vi "Polynomial Roots (DBL).vi"(10 "option":u16(ring)=1 items=["General", "Simple Classification", "Refinement", "Advanced Refinement"], 11 "P(x)":dbl[](array[numeric])) -> (0 "error":i32, 3 "Roots":cdb[](array[numeric]))   [LabVIEW 2020, in "NI_AALPro.lvlib"]
doc: "Finds the roots of polynomial <B>P(x)</B>. This VI removes leading coefficients of the polynomial that are equal to zero. Wire data to the <B>P(x)</B> input to determine the polymorphic instance to use or manually select the instance."
uses:
  NI_AALPro.lvlib
  <resource>/lvanlys.dll
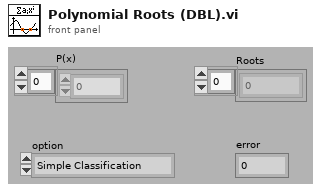
[diagram p1: front panel]
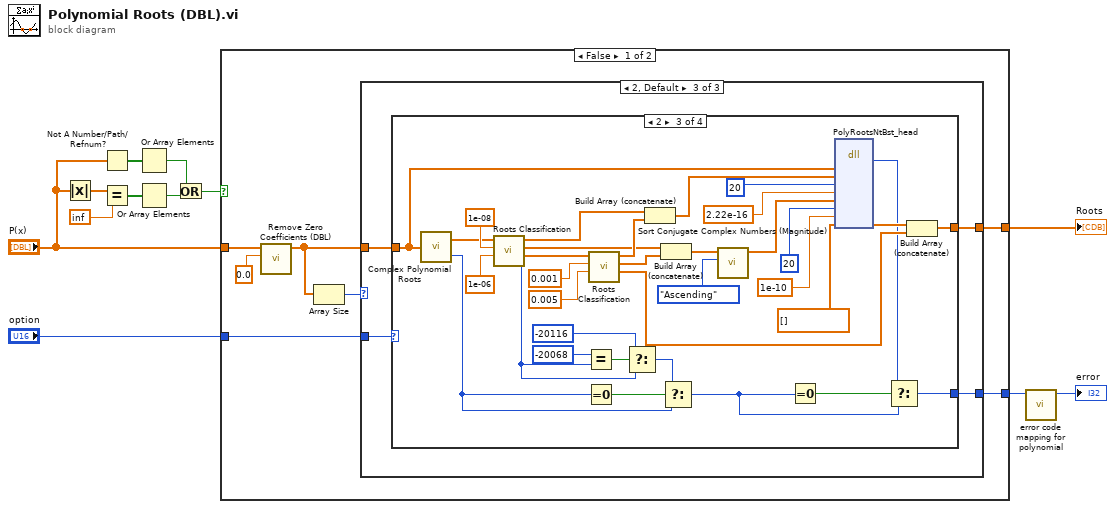
[diagram p0: block diagram]
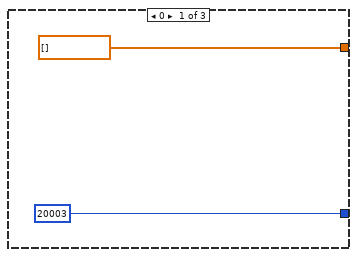
[diagram p2: hidden frame]
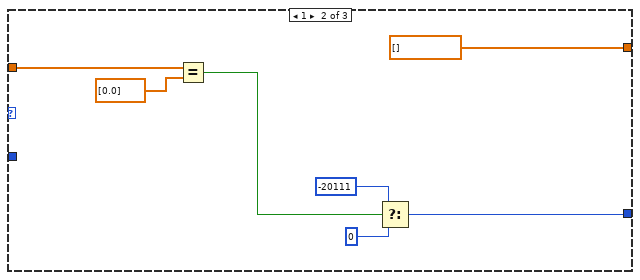
[diagram p3: hidden frame]
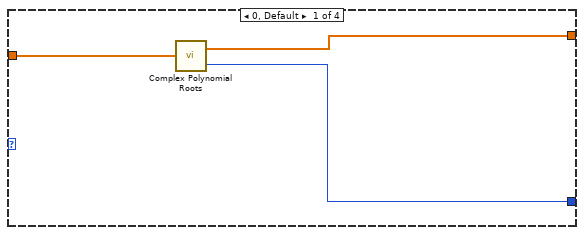
[diagram p4: hidden frame]
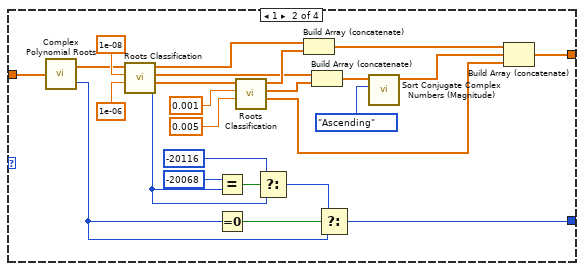
[diagram p5: hidden frame]
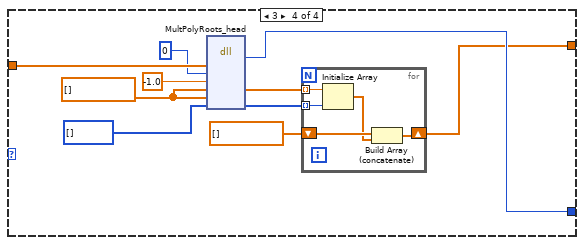
[diagram p6: hidden frame]
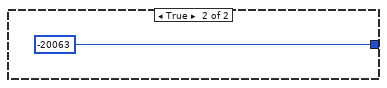
[diagram p7: hidden frame]
diagram:
  n1 = Absolute Value(x="P(x)") -> (abs(x)=w7:dbl[])
  n2 = Not A Number/Path/Refnum?(number/path/refnum="P(x)") -> (NaN/Path/Refnum?=w8:bool[])
  n3 = Equal?(x=w7, y=inf) -> (x = y?=w5:bool[])
  n4 = Or Array Elements(Boolean array=w8) -> (logical OR=w4:bool)
  n5 = Or Array Elements(Boolean array=w5) -> (logical OR=w3:bool)
  n6 = Or(x=w4, y=w3) -> (x .or. y?=w1:bool)
  n7 = case shown="False" w1 {
    tunnel: [w19 _] -> w12
    tunnel: "option" -> [w17 _]
    tunnel: [w16 -20063 ("error")] -> w10
    tunnel: "P(x)" -> [w14 _]
    frame False {
      n8 = call "Remove Zero Coefficients (DBL).vi"("threshold"=0.0, "P(x) In"=w14) -> ("P(x) Out"=w13:dbl[])  [unwired: 7 in, 2 out]
      n9 = Array Size(array=w13) -> (size(s)=w18:i32)
      n10 = case shown="2, Default" w18 {
        tunnel: w13 -> [_ w28 w29]
        tunnel: [20003 ("empty array") w23 w32] -> w16
        tunnel: [cdb[] [] cdb[] [] ("Polynomial Roots") w31] -> w19
        tunnel: w17 -> [_ _ w30]
        frame 0 {
        }
        frame 1 {
          n11 = Equal?(x=w28, y=dbl[] [0.0]) -> (x = y?=w25:bool)
          n12 = Select(t=-20111, s=w25, f=0) -> (s? t:f=w23:i32)
        }
        frame 2, Default {
          n13 = case shown="2" w30 {
            tunnel: w29 -> [w33 w41 w70 w104]
            tunnel: [w34 w42 w66 w102] -> w32
            tunnel: [w35 w50 w84 w101] -> w31
            frame 0, Default {
              n14 = call "Complex Polynomial Roots.vi"("Polynomial"=w33) -> ("Polynomial Roots"=w35:cdb[], "error"=w34:i32)
            }
            frame 1 {
              n15 = call "Complex Polynomial Roots.vi"("Polynomial"=w41) -> ("Polynomial Roots"=w48:cdb[], "error"=w43:i32)
              n16 = call "Roots Classification.vi"("tolerance for conjugate pair"=1e-06 ("threshold"), "tolerance for real roots"=1e-08 ("threshold"), "Roots"=w48) -> ("error"=w37:i32, "Pure Complex Roots"=w57:cdb[], "Complex Pair Roots"=w53:cdb[], "Real Roots"=w58:dbl[])  [unwired: 5 out]
              n17 = Equal?(x=-20068 ("y"), y=w37) -> (x = y?=w40:bool)
              n18 = Equal To 0?(x=w43) -> (x = 0?=w44:bool)
              n19 = call "Roots Classification.vi"("tolerance for conjugate pair"=0.005 ("tolerance for real roots"), "tolerance for real roots"=0.001, "Roots"=w57) -> ("Pure Complex Roots"=w49:cdb[], "Complex Pair Roots"=w52:cdb[], "Real Roots"=w54:dbl[])  [unwired: 6 out]
              n20 = Select(t=-20116, s=w40, f=w37) -> (s? t:f=w36:i32)
              n21 = Build Array (concatenate)(w58, w54) -> (w47:dbl[])
              n22 = Build Array (concatenate)(w53, w52) -> (w51:cdb[])
              n23 = Select(t=w36, s=w44, f=w43) -> (s? t:f=w42:i32)
              n24 = call "Sort Conjugate Complex Numbers (Magnitude).vi"("Order"=enum16{"Ascending", "Descending"}."Ascending", "Conjugate Complex Numbers"=w51) -> ("Sorted Conjugate Complex Numbers"=w46:cdb[])  [unwired: 9 out]
              n25 = Build Array (concatenate)(w47, w46, w49) -> (w50:cdb[])
            }
            frame 2 {
              n26 = call "Complex Polynomial Roots.vi"("Polynomial"=w70) -> ("Polynomial Roots"=w82:cdb[], "error"=w79:i32)
              n27 = call "Roots Classification.vi"("tolerance for conjugate pair"=1e-06 ("threshold"), "tolerance for real roots"=1e-08 ("threshold"), "Roots"=w82) -> ("error"=w64:i32, "Pure Complex Roots"=w91:cdb[], "Complex Pair Roots"=w87:cdb[], "Real Roots"=w92:dbl[])  [unwired: 5 out]
              n28 = Equal?(x=-20068 ("y"), y=w64) -> (x = y?=w65:bool)
              n29 = Equal To 0?(x=w79) -> (x = 0?=w80:bool)
              n30 = call "Roots Classification.vi"("tolerance for conjugate pair"=0.005 ("tolerance for real roots"), "tolerance for real roots"=0.001, "Roots"=w91) -> ("Pure Complex Roots"=w83:cdb[], "Complex Pair Roots"=w86:cdb[], "Real Roots"=w88:dbl[])  [unwired: 6 out]
              n31 = Select(t=-20116, s=w65, f=w64) -> (s? t:f=w62:i32)
              n32 = Build Array (concatenate)(w92, w88) -> (w78:dbl[])
              n33 = Build Array (concatenate)(w87, w86) -> (w85:cdb[])
              n34 = Select(t=w62, s=w80, f=w79) -> (s? t:f=w67:i32)
              n35 = call "Sort Conjugate Complex Numbers (Magnitude).vi"("Order"=enum16{"Ascending", "Descending"}."Ascending", "Conjugate Complex Numbers"=w85) -> ("Sorted Conjugate Complex Numbers"=w71:cdb[])  [unwired: 9 out]
              n36 = Equal To 0?(x=w67) -> (x = 0?=w69:bool)
              n37 = dll-call lib="C:/Program Files (x86)/National Instruments/LabVIEW 2020/resource/lvanlys.*" fn="PolyRootsNtBst_head"("poly"=w70, "FlRootsIn"=w78, "FlMaxIter"=20, "FlTol"=2.22e-16 ("2^x"), "CxRootsIn"=w71, "CxMaxIter"=20 ("FlMaxIter"), "CxTol"=1e-10 ("2^x"), "RootsOut"=cdb[] [] ("Roots")) -> ("return type"=w68:i32, "RootsOut"=w72:cdb[])  [unwired: 10 in, 2 out]
              n38 = Select(t=w68, s=w69, f=w67) -> (s? t:f=w66:i32)
              n39 = Build Array (concatenate)(w72, w83) -> (w84:cdb[])
            }
            frame 3 {
              w98 = cdb[] []
              n40 = dll-call lib="C:/Program Files (x86)/National Instruments/LabVIEW 2020/resource/lvanlys.*" fn="MultPolyRoots_head"("pH"=w104, "alg2"=0, "tol"=-1.0, "appRootH"=w98, "rootH"=w98, "multH"=i32[] []) -> ("return type"=w102:i32, "appRootH"=w95:cdb[], "multH"=w99:i32[])  [unwired: 6 in, 3 out]
              n41 = for {
                tunnel: w95 -> [w109] mode=indexing
                tunnel: w99 -> [w108] mode=indexing
                shift-right: [w105] -> w101
                shift-left: cdb[] [] -> [w107]
                n42 = Initialize Array(w109, w108) -> (w106:cdb[])
                n43 = Build Array (concatenate)(w107, w106) -> (w105:cdb[])
              }
            }
          }
        }
      }
    }
    frame True {
    }
  }
  "Roots" <- w12
  n44 = call "error code mapping for polynomial.vi"("error in"=w10) -> ("error out"=→"error":i32)  [unwired: 10 out]
